vi "close.vi"(8 "error in (no error)":errorcluster, 11 "DesktopModbus in":refnum<class "DesktopModbus.lvclass">) -> (0 "error out":errorcluster, 3 "DesktopModbus out":refnum<class "DesktopModbus.lvclass">)   [LabVIEW 2016, in "DesktopModbus.lvclass"]
uses:
  DesktopModbus.lvclass
  DesktopModbus.lvclass/DesktopModbus.ctl
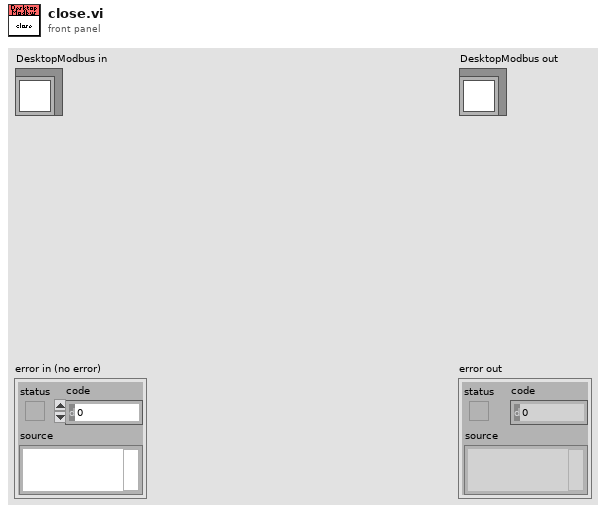
[diagram p1: front panel]
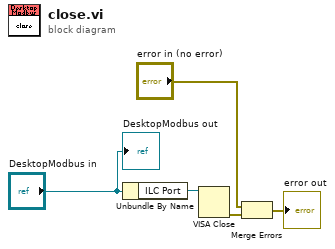
[diagram p0: block diagram]
diagram:
  n1 = Unbundle By Name("DesktopModbus in") -> ("ILC Port"=w5:refnum<visa-resource-name>)
  n2 = VISA Close(VISA resource name=w5) -> (error out=w4:errorcluster)  [unwired: 1 in]
  n3 = Merge Errors("error in (no error)", w4) -> (→"error out":errorcluster)
  "DesktopModbus out" <- "DesktopModbus in"
